vi "SCM4 User Client.vi"() -> ()   [LabVIEW 2020]
doc: "Author: Scott Hannahs <sth@magnet.fsu.edu>\nCopyright 2018 Florida State University, All rights reserved."
uses:
  SCM4 Interlock LV20/RT SubVIs/RT System Auth Level.ctl
  SCM4 Interlock LV20/RT SubVIs/PS Action Control.ctl
  <vilib>/Utility/miscctls.llb/LVOffsetAndMultiplierTypeDef.ctl
  SCM4 Interlock LV20/RT SubVIs/Interlock RT FPGA Status Info.ctl
  SCM4 Interlock LV20/FPGA SubVIs/FPGA Crowbar State.ctl
  SCM4 Interlock LV20/RT SubVIs/Switch Box Status.ctl
  SubVIs/Interlock 32T Net Client Globals.vi
  TCP Functions/TCP Read Length and Value (STR).vi
  <vilib>/Utility/miscctls.llb/LVRectTypeDef.ctl
  <vilib>/Utility/miscctls.llb/LVPointTypeDef.ctl
panel:
  out "# Clients":u32
  out "Currents":dbl[][](graph)
  in  "Client Loop Time (mS)":u32=100
  out "Start DateStamp":timestamp format="%<%H:%M:%S%4u\n%Y/%m/%d>T"
  out "Version RT System":string
  out "Version FPGA":string
  in  "Password":string
  out "Authorized":T1
  in  "Slew rate [T/min]":dbl format="%.3g"
  out "Field [T]":dbl format="%.5f"
  in  "Setpoint [T]":dbl format="%.6g"
  in  "PS Action":T2=enum."Hold"
  out "Version":string
  in  "stop":bool
  # "NHMFL 32T User Control"
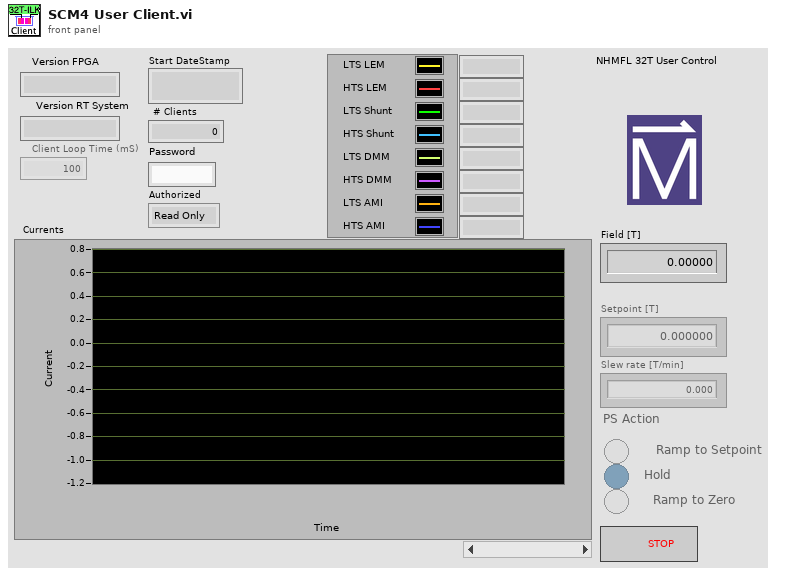
[diagram p1: front panel]
types:
  T1 = typedef "RT System Auth Level.ctl" = enum16{"Read Only", "User", "Operator", "Admin"}
  T2 = typedef "PS Action Control.ctl" = enum32{"Ramp to Setpoint", "Hold", "Ramp to Zero"}
  T3 = enum8{"Enabled", "Disabled", "Disabled and Grayed Out"}
  T4 = typedef "LVPointTypeDef.ctl" = cluster{"Horizontal":i16, "Vertical":i16}
  T5 = typedef "LVRectTypeDef.ctl" = cluster{"Left":i16, "Top":i16, "Right":i16, "Bottom":i16}
  T6 = typedef "LVOffsetAndMultiplierTypeDef.ctl" = cluster{"Offset":dbl, "Multiplier":dbl}
  T7 = enum16{"Standard", "Buffered", "CRLF", "Immediate"}
  T8 = typedef "Interlock RT FPGA Status Info.ctl" = cluster{"Authorized":T1, "# Clients":u32, "Chassis Temperature":fxp<+/-,16,14>, "Secondary QD Time Constant":enum16{"2000 mS", "1000 mS", "200 mS", "50 mS"}, "Crowbar Latch State":T9, "Crowbar Reset Countdown Length (ms)":i32, "Crowbar Reset Countdown":i32, "Ramp To Zero Fault":u16, "Crowbar Fault":u16, "Protection Logic V":dbl, "Quench Loop":dbl, "HTS LEM":dbl, "HTS Shunt":dbl, "LTS LEM":dbl, "LTS Shunt":dbl, "Ramp To Zero":bool, "2 Crowbar Reset Key":bool, "7 Crowbar LED":bool, "15 Close Switch Box 2 Contactor":bool, "HTS Voltage":dbl, "LTS Voltage":dbl, "PS Check Loop Ticks":u32, "Main Loop Ticks":u32, "DAQ Loop Ticks":u32, "WDT Loop Ticks":u32, "LHe Level 1":dbl, "LHe Level 2":dbl, "HTS DMM":dbl, "LTS DMM":dbl, "HTS AMI430":dbl, "LTS AMI430":dbl, "Battery Monitor Alarm":bool, "Switch Box Status":T10, "PS Action":T2, "Setpoint [T]":dbl, "Field [T]":dbl, "Slew rate [T/min]":dbl, "Recorded error":errorcluster, "Last Batt Comm":timestamp, "Batt Alarm Text":string, "PS Comm Time (ms)":u32, "DMM Comm Time (ms)":u32}
  T9 = typedef "FPGA Crowbar State.ctl" = enum16{"Run", "Crowbar", "Reset Countdown"}
  T10 = typedef "Switch Box Status.ctl" = cluster{"Battery Voltage":dbl, "SwBox 1 Contactor V":dbl, "SwBox 2 Contactor V":dbl, "Battery Ground V":dbl}
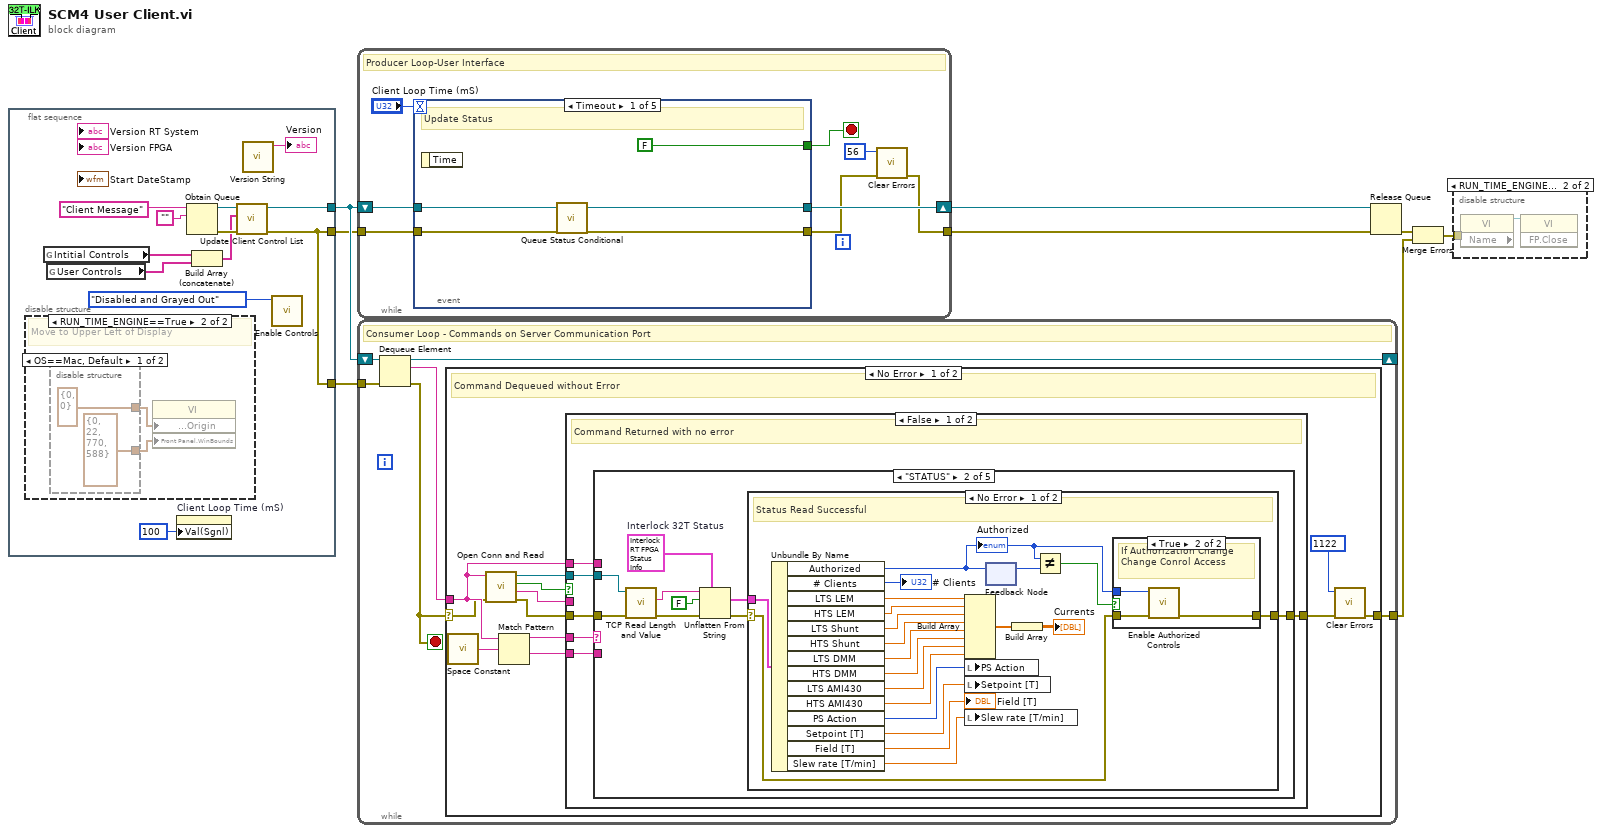
[diagram p0: block diagram]
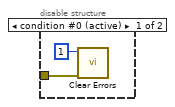
[diagram p2: hidden frame]
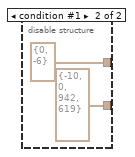
[diagram p4: hidden frame]
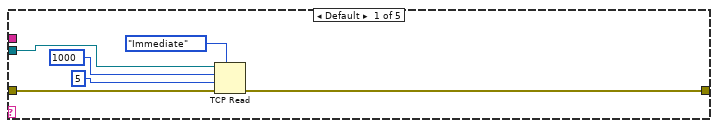
[diagram p5: hidden frame]
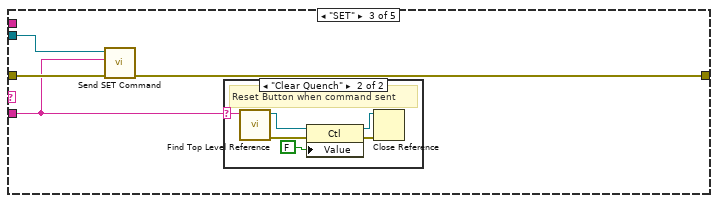
[diagram p8: hidden frame]
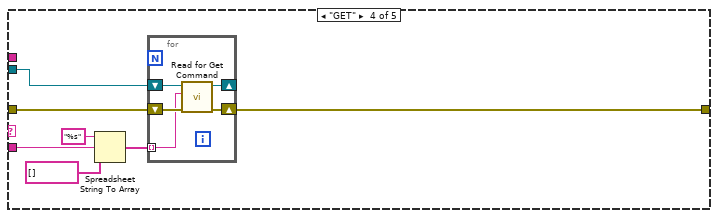
[diagram p10: hidden frame]
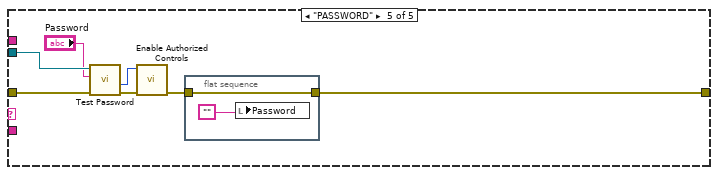
[diagram p11: hidden frame]
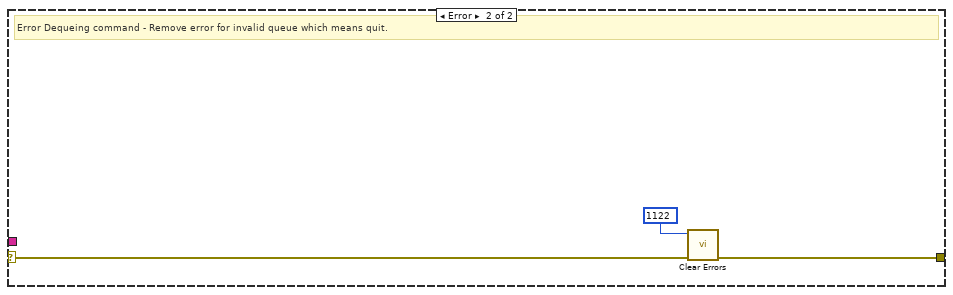
[diagram p13: hidden frame]
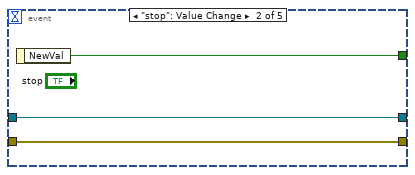
[diagram p14: hidden frame]
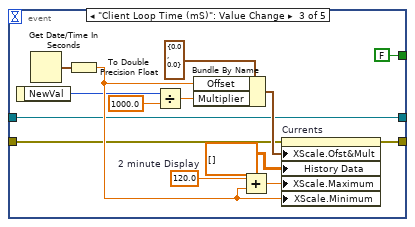
[diagram p15: hidden frame]
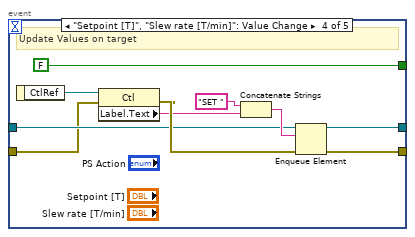
[diagram p16: hidden frame]
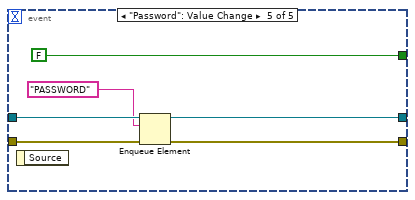
[diagram p17: hidden frame]
diagram:
  n1 = flat-sequence {
    tunnel: [w20] -> w6
    tunnel: [w10] -> w3
    tunnel: [w10] -> w1
    frame #0 {
      n2 = disable-structure shown="RUN_TIME_ENGINE==True" {
        frame condition #0 (active) {
        }
        frame condition #1 {
          # "Move to Upper Left of Display"
          n3 = disable-structure shown="OS==Mac, Default" {
            disable-tunnel: [T5 {"Left"=0, "Top"=22, "Right"=770, "Bottom"=588} ("Front Panel Window:Window Bounds") T5 {"Left"=-10, "Top"=0, "Right"=942, "Bottom"=619} ("Front Panel Window:Window Bounds")] -> w22
            disable-tunnel: [T4 {"Horizontal"=0, "Vertical"=0} ("Front Panel Window:Origin") T4 {"Horizontal"=0, "Vertical"=-6} ("Front Panel Window:Origin")] -> w21
            frame condition #0 (active) {
            }
            frame condition #1 {
            }
          }
          n4 = property class="VI"("Front Panel Window:Origin"=w21, "Front Panel.WinBounds"=w22) -> ()  [unwired: 2 in, 2 out]
        }
      }
      n5 = global read "Interlock 32T Net Client Globals.vi" "Intitial Controls"() -> (w12:string[])
      n6 = global read "Interlock 32T Net Client Globals.vi" "User Controls"() -> (w11:string[])
      n7 = property on="Client Loop Time (mS)" class="DigNum (strict)"("Val(Sgnl)"=u32 100 ("Value (Signaling)")) -> ()  [unwired: 2 in, 2 out]
      n8 = Obtain Queue(name (unnamed)="Client Message", element data type="") -> (queue out=w17:refnum<queue>, error out=w16:errorcluster)  [unwired: 3 in, 1 out]
      n9 = Build Array (concatenate)(w12, w11) -> (w14:string[])
      n10 = call "Update Client Control List.vi"("error in (no error)"=w16, "Array"=w14, "Queue in"=w17) -> ("error out"=w10:errorcluster, "Queue out"=w20:refnum<queue>)  [unwired: 6 in, 1 out]
      n11 = call "Version String.vi"() -> ("String"=→"Version":string)  [unwired: 10 in, 1 out]
      n12 = call "Enable Controls.vi"("Enable Disable"=T3."Disabled and Grayed Out") -> ()  [unwired: 10 in, 1 out]
    }
  }
  n13 = while {
    tunnel: w3 -> [w28]
    tunnel: [w29] -> w5
    shift-right: [w32] -> w8
    shift-left: w6 -> [w33]
    stop <- w30 stop-if-true
    # "Producer Loop-User Interface"
    n14 = event shown="[0] Timeout" {
      selector: _ -> [_ _ _ _ _]
      dyn-events: _ -> [_ _ _ _ _]
      timeout: "Client Loop Time (mS)" -> [_ _ _ _ _]
      tunnel: w28 -> [w38 w42 w43 w61 w71]
      tunnel: [w36 w42 w44 w59 w70] -> w31
      tunnel: [w35 w41 w46 w58 w69] -> w32
      tunnel: w33 -> [w37 w41 w46 w62 w72]
      tunnel: [FALSE ("NewVal") w40 FALSE ("NewVal") FALSE ("NewVal") FALSE ("NewVal")] -> w30
      event Timeout {
        # "Update Status"
        n15 = event-data() -> ()  [unwired: 1 in, 1 out]
        n16 = call "Queue Status Conditional.vi"("error in (no error)"=w38, "Queue in"=w37) -> ("error out"=w36:errorcluster, "Queue out"=w35:refnum<queue>)  [unwired: 8 in]
      }
      event "stop": Value Change {
        n17 = event-data() -> ("NewVal"=w40:bool)  [unwired: 1 in]
      }
      event "Client Loop Time (mS)": Value Change {
        w51 = 120.0  # 2 minute Display
        n18 = event-data() -> ("NewVal"=w47:u32)  [unwired: 1 in]
        n19 = Get Date/Time In Seconds() -> (seconds since 1Jan1904=w52:timestamp)
        n20 = To Double Precision Float(number=w52) -> (double precision float=w56:dbl)
        n21 = Divide(x=w47, y=1000.0) -> (x/y=w54:dbl)
        n22 = Bundle By Name(cluster=T6 {"Offset"=0.0, "Multiplier"=0.0} ("X Scale.Offset and Multiplier"), "Offset"=w56, "Multiplier"=w54) -> (w53:T6)
        n23 = Add(x=w51, y=w56) -> (x+y=w55:dbl)
        n24 = property on="Currents" class="WFChart (strict)"(error in=w43, "XScale.Ofst&Mult"=w53, "History Data"=dbl[][] [], "XScale.Maximum"=w55, "XScale.Minimum"=w56) -> (error out=w44:errorcluster)  [unwired: 1 in, 1 out]
      }
      event "Setpoint [T]", "Slew rate [T/min]": Value Change {
        # "Update Values on target"
        n25 = event-data() -> ("CtlRef"=w66:refnum<vi>)  [unwired: 1 in]
        n26 = property class="Ctl"(reference=w66, error in=w61) -> (error out=w64:errorcluster, "Label.Text"=w60:string)  [unwired: 1 out]
        n27 = Concatenate Strings("SET " ("string"), w60) -> (w63:string)
        n28 = Enqueue Element(queue=w62, element=w63, error in (no error)=w64) -> (queue out=w58:refnum<queue>, error out=w59:errorcluster)  [unwired: 1 in, 1 out]
      }
      event "Password": Value Change {
        n29 = event-data() -> ()  [unwired: 1 in, 1 out]
        n30 = Enqueue Element(queue=w72, element="PASSWORD" ("string"), error in (no error)=w71) -> (queue out=w69:refnum<queue>, error out=w70:errorcluster)  [unwired: 1 in, 1 out]
      }
    }
    n31 = call <vilib>:"Clear Errors.vi"("error in (no error)"=w31, "specific error code to clear (0: all)"=56) -> ("error out"=w29:errorcluster)  [unwired: 4 in, 1 out]
  }
  n32 = while {
    shift-right: [w76] -> _
    shift-left: w6 -> [w78]
    tunnel: w1 -> [w77]
    tunnel: [w73] -> w4
    stop <- w74 stop-if-true
    # "Consumer Loop - Commands on Server Communication Port"
    n33 = Dequeue Element(queue=w78, error in (no error)=w77) -> (queue out=w76:refnum<queue>, element=w75:string, error out=w74:errorcluster)  [unwired: 1 in, 1 out]
    n34 = case shown="No Error" w74 {
      selector: w74 -> [w82 w172]
      tunnel: [w80 w171] -> w73
      tunnel: w75 -> [w86 _]
      frame No Error {
        # "Command Dequeued without Error"
        n35 = call <vilib>:"Space Constant.vi"() -> ("String"=w84:string)
        n36 = call "Open Conn and Read.vi"("error in (no error)"=w82, "String"=w86) -> ("error out"=w88:errorcluster, "Returned String"=w90:string, "Returned Error"=w87:bool, "TCP Network Connection out"=w89:refnum<k5>)  [unwired: 6 in]
        n37 = Match Pattern(string=w86, regular expression=w84) -> (before substring=w85:string, after substring=w83:string)  [unwired: 1 in, 2 out]
        n38 = case shown="False" w87 {
          tunnel: [w96 w169] -> w79
          tunnel: w90 -> [_ _]
          tunnel: w89 -> [w95 _]
          tunnel: w88 -> [w94 w169]
          tunnel: w86 -> [w93 _]
          tunnel: w85 -> [w92 _]
          tunnel: w83 -> [w91 _]
          frame False {
            # "Command Returned with no error"
            n39 = case shown="\"STATUS\"" w92 {
              tunnel: [w97 w103 w140 w148 w163] -> w96
              tunnel: w94 -> [w99 w110 w141 w154 w166]
              tunnel: w95 -> [w98 w109 w139 w150 w165]
              tunnel: w93 -> [_ _ _ _ _]
              tunnel: w91 -> [_ _ w138 w149 _]
              frame Default {
                n40 = TCP Read(connection ID=w98, bytes to read=1000, error in (no error)=w99, 7:T7."Immediate" ("mode (standard)"), 9:5 ("timeout ms (25000)")) -> (error out=w97:errorcluster)  [unwired: 2 out]
              }
              frame "STATUS" {
                w105 = T8 {"Authorized"=enum."Read Only", "# Clients"=0, "Chassis Temperature"=0.0, "Secondary QD Time Constant"=enum."2000 mS", "Crowbar Latch State"=enum."Run", "Crowbar Reset Countdown Length (ms)"=0, "Crowbar Reset Countdown"=0, "Ramp To Zero Fault"=0, "Crowbar Fault"=0, "Protection Logic V"=0.0, "Quench Loop"=0.0, "HTS LEM"=0.0, "HTS Shunt"=0.0, "LTS LEM"=0.0, "LTS Shunt"=0.0, "Ramp To Zero"=FALSE, "2 Crowbar Reset Key"=FALSE, "7 Crowbar LED"=FALSE, "15 Close Switch Box 2 Contactor"=FALSE, "HTS Voltage"=0.0, "LTS Voltage"=0.0, "PS Check Loop Ticks"=0, "Main Loop Ticks"=0, "DAQ Loop Ticks"=0, "WDT Loop Ticks"=0, "LHe Level 1"=2.148782730102539, "LHe Level 2"=3.334085464477539, "HTS DMM"=0.0, "LTS DMM"=0.0, "HTS AMI430"=0.0, "LTS AMI430"=0.0, "Battery Monitor Alarm"=FALSE, "Switch Box Status"={"Battery Voltage"=0.0, "SwBox 1 Contactor V"=0.0, "SwBox 2 Contactor V"=0.0, "Battery Ground V"=0.0}, "PS Action"=enum."Ramp to Zero", "Setpoint [T]"=0.0, "Field [T]"=0.0, "Slew rate [T/min]"=0.01, "Recorded error"={"status"=FALSE, "code"=0, "source"=""}, "Last Batt Comm"=timestamp(0 s since 1904-01-01), "Batt Alarm Text"="", "PS Comm Time (ms)"=0, "DMM Comm Time (ms)"=0}  # Interlock 32T Status
                n41 = call-poly "TCP Read Length and Value.vi"("error in (no error)"=w110, "TCP Network Connection in"=w109) -> ("error out"=w111:errorcluster, "Output"=w107:string)  [unwired: 7 in, 1 out]
                n42 = Unflatten From String(type=w105, binary string=w107, data includes array or string size? (T)=FALSE, error in (no error)=w111) -> (value=w108:T8, error out=w104:errorcluster)  [unwired: 1 in, 1 out]
                n43 = case shown="No Error" w104 {
                  selector: w104 -> [w128 w137]
                  tunnel: w108 -> [w132 _]
                  tunnel: [w127 w137] -> w103
                  frame No Error {
                    # "Status Read Successful"
                    n44 = Unbundle By Name(w132) -> ("Authorized"=w129:T1, "# Clients"=→"# Clients":u32, "LTS LEM"=w124:dbl, "HTS LEM"=w123:dbl, "LTS Shunt"=w121:dbl, "HTS Shunt"=w120:dbl, "LTS DMM"=w115:dbl, "HTS DMM"=w114:dbl, "LTS AMI430"=w113:dbl, "HTS AMI430"=w112:dbl, "PS Action"=w119:T2, "Setpoint [T]"=w118:dbl, "Field [T]"=→"Field [T]":dbl, "Slew rate [T/min]"=w116:dbl)
                    "Authorized" <- w129
                    n45 = Build Array(w124, w123, w121, w120, w115, w114, w113, w112) -> (w126:dbl[])
                    n46 = local write "PS Action"(w119) -> ()
                    n47 = local write "Setpoint [T]"(w118) -> ()
                    n48 = local write "Slew rate [T/min]"(w116) -> ()
                    n49 = feedback-in #1(w129) -> ()
                    n50 = feedback #1() -> (w131:T1)  [unwired: 1 in]
                    n51 = Build Array(w126) -> (→"Currents":dbl[][])
                    n52 = Not Equal?(x=w129, y=w131) -> (x != y?=w130:bool)
                    n53 = case shown="True" w130 {
                      tunnel: w129 -> [_ w136]
                      tunnel: w128 -> [w133 w135]
                      tunnel: [w133 w134] -> w127
                      frame False {
                      }
                      frame True {
                        # "If Authorization Change\nChange Conrol Access"
                        n54 = call "Enable Authorized Controls.vi"("error in (no error)"=w135, "Authorized"=w136) -> ("error out"=w134:errorcluster)  [unwired: 9 in]
                      }
                    }
                  }
                  frame Error {
                    # "Status Not Read"
                  }
                }
              }
              frame "SET" {
                n55 = call "Send SET Command.vi"("error in (no error)"=w141, "Control Name"=w138, "TCP Network Connection in"=w139) -> ("error out"=w140:errorcluster)  [unwired: 8 in]
                n56 = case shown="\"Clear Quench\"" w138 {
                  selector: w138 -> [_ w147]
                  frame Default {
                  }
                  frame "Clear Quench" {
                    # "Reset Button when command sent"
                    n57 = call "Find Top Level Reference.vi"("String"=w147) -> ("error out"=w142:errorcluster, "Ctl Refnum"=w146:refnum<vi>)  [unwired: 9 in]
                    n58 = property class="Ctl"(reference=w146, error in=w142, "Value"=FALSE) -> (reference out=w143:refnum<vi>, error out=w144:errorcluster)
                    n59 = Close Reference(reference=w143, error in (no error)=w144) -> ()  [unwired: 1 out]
                  }
                }
              }
              frame "GET" {
                n60 = Spreadsheet String To Array(format string="%s", spreadsheet string=w149, array type (2D Dbl)=string[] []) -> (array=w153:string[])  [unwired: 1 in]
                n61 = for {
                  tunnel: w153 -> [w156] mode=indexing
                  shift-right: [w157] -> w148
                  shift-left: w154 -> [w158]
                  shift-right: [w155] -> _
                  shift-left: w150 -> [w159]
                  n62 = call "Read for Get Command.vi"("error in (no error)"=w158, "Control Name"=w156, "TCP Network Connection in"=w159) -> ("error out"=w157:errorcluster, "TCP Network Connection out"=w155:refnum<k5>)  [unwired: 7 in]
                }
              }
              frame "PASSWORD" {
                n63 = call "Test Password.vi"("error in (no error)"=w166, "String"="Password", "TCP Network Connection in"=w165) -> ("error out"=w160:errorcluster, "Authorized"=w162:T1)  [unwired: 6 in, 1 out]
                n64 = call "Enable Authorized Controls.vi"("error in (no error)"=w160, "Authorized"=w162) -> ("error out"=w161:errorcluster)  [unwired: 9 in]
                n65 = flat-sequence {
                  tunnel: w161 -> [w168]
                  tunnel: [w168] -> w163
                  frame #0 {
                    n66 = local write "Password"("") -> ()
                  }
                }
              }
            }
          }
          frame True {
          }
        }
        n67 = call <vilib>:"Clear Errors.vi"("error in (no error)"=w79, "specific error code to clear (0: all)"=1122) -> ("error out"=w80:errorcluster)  [unwired: 4 in, 1 out]
      }
      frame Error {
        # "Error Dequeing command - Remove error for invalid queue which means quit."
        n68 = call <vilib>:"Clear Errors.vi"("error in (no error)"=w172, "specific error code to clear (0: all)"=1122) -> ("error out"=w171:errorcluster)  [unwired: 4 in, 1 out]
      }
    }
  }
  n69 = Release Queue(queue=w8, error in (no error)=w5) -> (error out=w7:errorcluster)  [unwired: 1 in, 2 out]
  n70 = Merge Errors(w7, w4) -> (w2:errorcluster)
  n71 = disable-structure shown="RUN_TIME_ENGINE==True" {
    disable-tunnel: w2 -> [w174 _]
    frame condition #0 (active) {
      n72 = call <vilib>:"Clear Errors.vi"("error in (no error)"=w174, "specific error code to clear (0: all)"=1) -> ()  [unwired: 4 in, 2 out]
    }
    frame condition #1 {
      n73 = property class="VI" props=["Name"]() -> (reference out=w175:refnum<vi>)  [unwired: 2 in, 2 out]
      n74 = invoke class="VI" method="FP.Close"(reference=w175) -> ()  [unwired: 2 in, 3 out]
    }
  }
